vi "checkBeginNormalDefensiveWithDuelistPlay.vi"(10 "Game":refnum<class "Game.lvclass">, 11 "NormalDefensiveWithDuelistPlay in":refnum<class "NormalDefensiveWithDuelistPlay.lvclass">) -> (2 "Duelist?":bool, 3 "NormalDefensiveWithDuelistPlay out":refnum<class "NormalDefensiveWithDuelistPlay.lvclass">)   [LabVIEW 2023, in "NormalDefensiveWithDuelistPlay.lvclass"]
uses:
  NormalDefensiveWithDuelistPlay.lvclass
  Game_class/Game.lvclass
  Utilities_class/Utilities.lvclass
  Referee_class/command_interpreted.ctl
  Game_class/Game.lvclass/Game.ctl
  Ball_class/Ball.lvclass/Ball.ctl
  Object_class/Object.lvclass/Object.ctl
  Team_class/Team.lvclass/Team.ctl
  Events_class/Events.lvclass/Events.ctl
  Referee_class/Referee.lvclass/Referee.ctl
  Parameters_class/Parameters.lvclass/Parameters.ctl
  Game_class/Read Parameters.lvclass.vi
  Parameters_class/Read AttakingOurselves.vi
  Game_class/Read EventsRef.vi
  Game_class/Read Referee.vi
  Game_class/Read EnemyRef.vi
  Game_class/Read BallRef.vi
  Object_class/Read x.vi
  Object_class/Read y.vi
  Team_class/Read RobotRef.vi
  Referee_class/Read command_interpreted.vi
  Events_class/Read ball_inside_our_goalie_area.vi
  Game_class/Read OffensiveTeam.vi
  Game_class/Read FieldRef.vi
  Game_class/Read DefensiveTeam.vi
  Ball_class/Read v_x.vi
  Ball_class/Read v_y.vi
  Ball_class/Ball.lvclass
  C:/Users/roboi/Downloads/VSS_AI-Larc2023 - Copia (2)/Object_class/Object.lvclass
  Enemy_class/Enemy.lvclass
  C:/Users/roboi/Downloads/VSS_AI-Larc2023 - Copia (2)/Team_class/Team.lvclass
  Ally_class/Ally.lvclass
  Robot_class/Robot.lvclass
  Events_class/Events.lvclass
  Referee_class/Referee.lvclass
  Parameters_class/Parameters.lvclass
  Field_class/Field.lvclass
panel:
  out "error out":errorcluster
  in  "error in (no error)":errorcluster
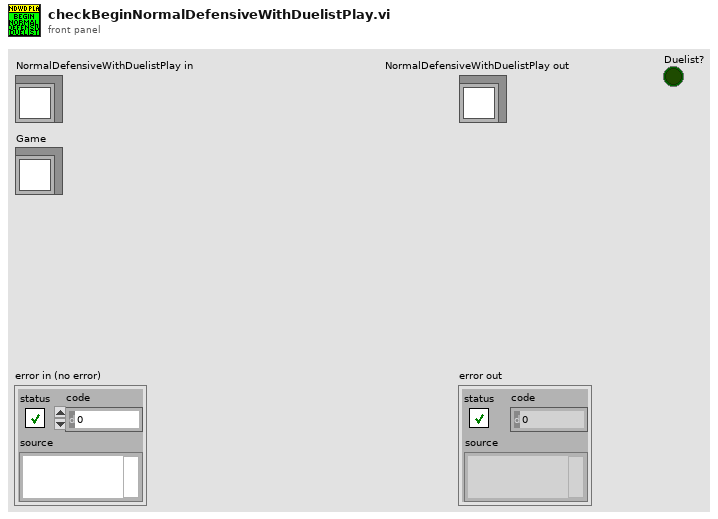
[diagram p1: front panel]
types:
  T1 = typedef "command_interpreted.ctl" = enum16{"Goal Ally", "Goal Enemy", "Ball Placement Enemy", "Ball Placement Ally", "Normal Half Time", "Extra Time  Break", "Extra Half Time", "None", "Post Game", "PKA Normal Start", "Prepare Kickoff Ally", "PKE Normal Start", "Prepare Kickoff Enemy", "Force Start", "Halt", "Timeout", "Prepare Penalty Ally", "Prepare Penalty Enemy", "PPA NormalStart", "PPE Normal Start", "Indirect Free Ally", "Direct Free Enemy", "Direct Free Ally", "Indirect Free Enemy", "Stop"}
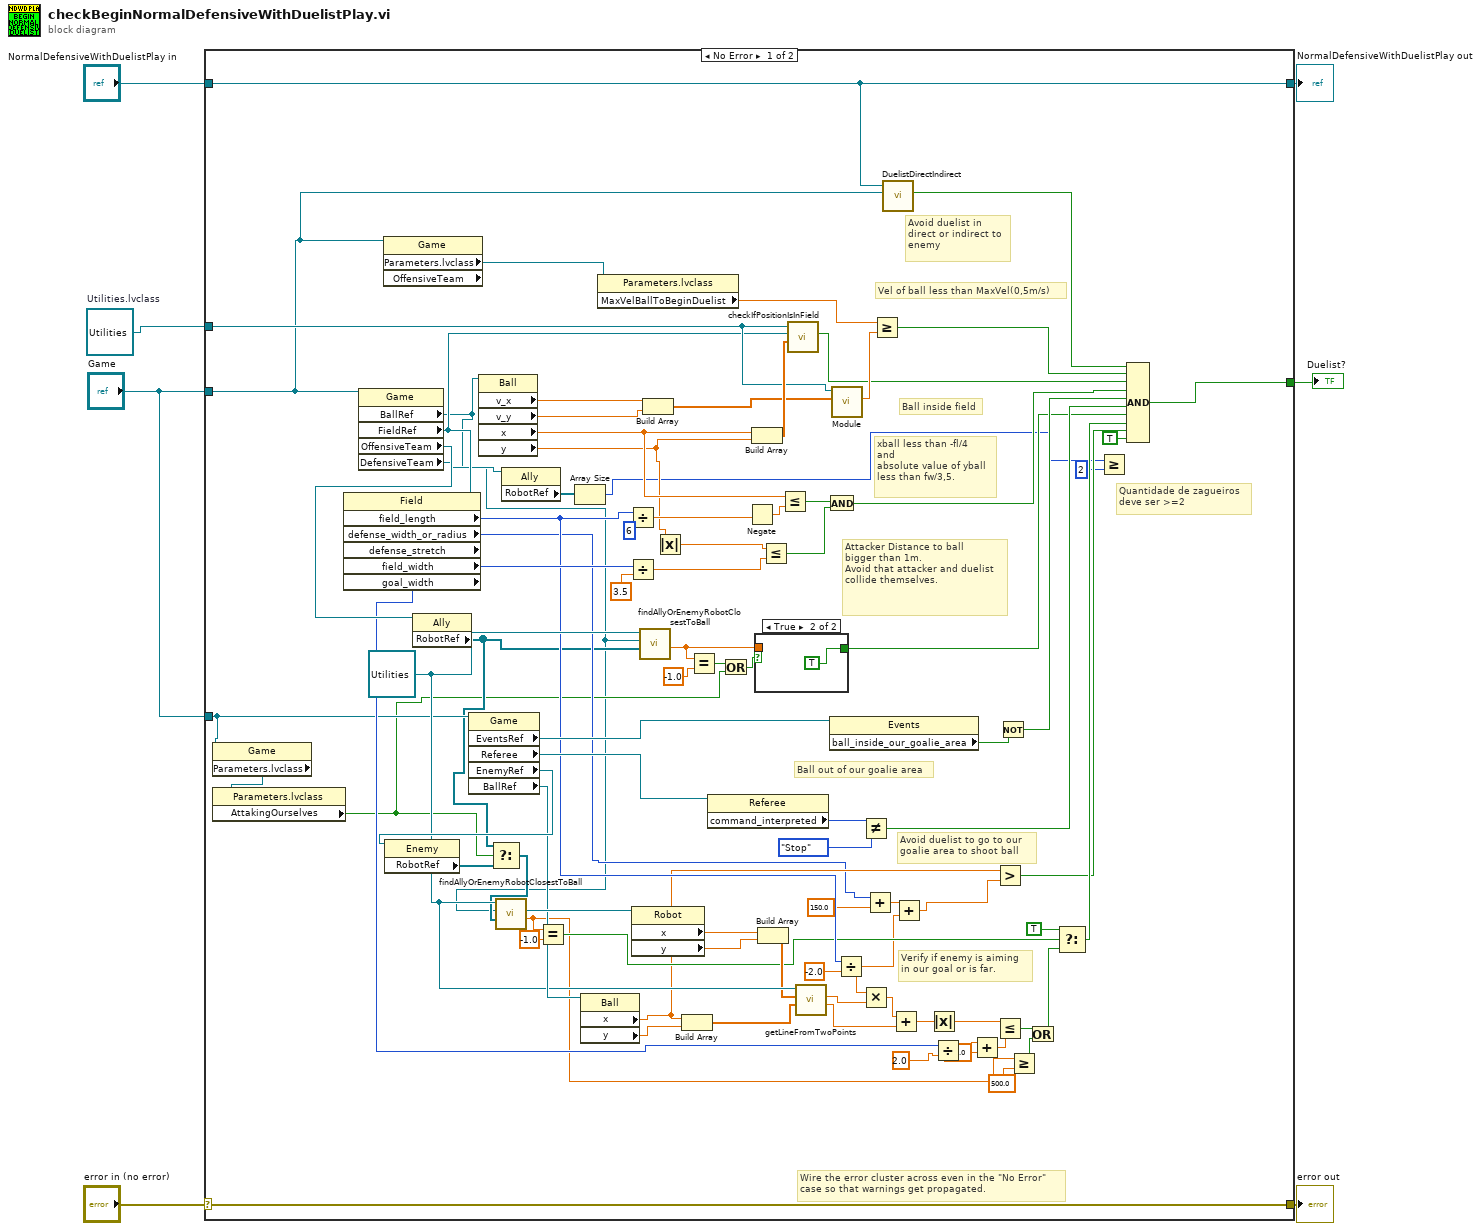
[diagram p0: block diagram]
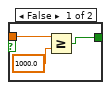
[diagram p2: hidden frame]
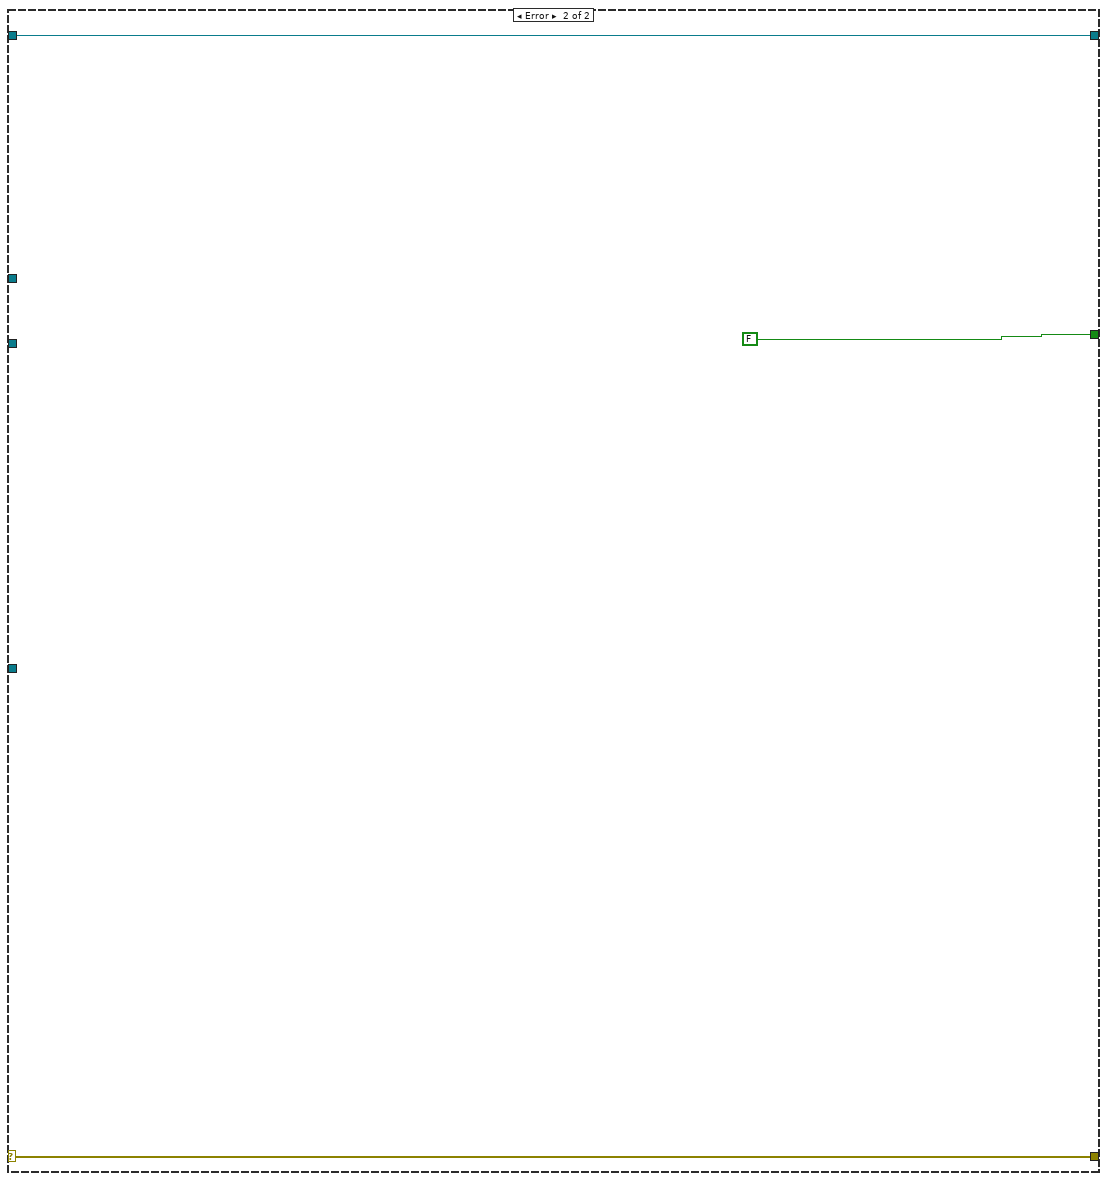
[diagram p3: hidden frame]
diagram:
  w3 = refnum<class "Utilities.lvclass"> refnum  # Utilities.lvclass
  n1 = case shown="No Error" "error in (no error)" {
    selector: "error in (no error)" -> [w97 w104]
    tunnel: [w97 w104] -> w6
    tunnel: [w83 w103] -> w4
    tunnel: "NormalDefensiveWithDuelistPlay in" -> [w83 w103]
    tunnel: w3 -> [w88 _]
    tunnel: "Game" -> [w82 _]
    tunnel: [w84 FALSE] -> w2
    tunnel: "Game" -> [w29 _]
    frame No Error {
      w54 = refnum<class "Utilities.lvclass"> refnum ("Utilities in")
      # "Quantidade de zagueiros\ndeve ser >=2"
      # "Avoid duelist to go to our\ngoalie area to shoot ball"
      # "Avoid duelist in\ndirect or indirect to\nenemy"
      # "Verify if enemy is aiming\nin our goal or is far."
      # "Attacker Distance to ball\nbigger than 1m. \nAvoid that attacker and duelist\ncollide themselves."
      # "Vel of ball less than MaxVel(0,5m/s)"
      # "Ball inside field"
      # "xball less than -fl/4\nand \nabsolute value of yball\nless than fw/3,5."
      # "Ball out of our goalie area"
      # "Wire the error cluster across even in the \"No Error\"\ncase so that warnings get propagated."
      n2 = property class="Game"(reference=w29) -> ("Parameters.lvclass"=w28:refnum<class "Parameters.lvclass">)  [unwired: 1 in, 2 out]
      n3 = property class="Parameters.lvclass"(reference=w28) -> ("AttakingOurselves"=w23:bool)  [unwired: 1 in, 2 out]
      n4 = property class="Game"(reference=w82) -> ("BallRef"=w8:refnum<class "Ball.lvclass">, "FieldRef"=w14:refnum<class "Field.lvclass">, "OffensiveTeam"=w63:refnum<class "Ally.lvclass">, "DefensiveTeam"=w13:refnum<class "Ally.lvclass">)  [unwired: 1 in, 2 out]
      n5 = property class="Field" props=["field_length", "defense_width_or_radius", "defense_stretch", "field_width", "goal_width"](reference=w14) -> ("field_length"=w48:i32, "defense_width_or_radius"=w33:i32, "field_width"=w67:i32, "goal_width"=w44:i32)  [unwired: 1 in, 3 out]
      n6 = property class="Game" props=["Parameters.lvclass", "OffensiveTeam"](reference=w82) -> ("Parameters.lvclass"=w94:refnum<class "Parameters.lvclass">)  [unwired: 1 in, 3 out]
      n7 = property class="Ally"(reference=w63) -> ("RobotRef"=w26:refnum<class "Robot.lvclass">[])  [unwired: 1 in, 2 out]
      n8 = property class="Game"(reference=w29) -> ("EventsRef"=w80:refnum<class "Events.lvclass">, "Referee"=w79:refnum<class "Referee.lvclass">, "EnemyRef"=w59:refnum<class "Enemy.lvclass">, "BallRef"=w56:refnum<class "Ball.lvclass">)  [unwired: 1 in, 2 out]
      n9 = property class="Enemy"(reference=w59) -> ("RobotRef"=w27:refnum<class "Robot.lvclass">[])  [unwired: 1 in, 2 out]
      n10 = property class="Ball"(reference=w8) -> ("v_x"=w93:dbl, "v_y"=w92:dbl, "x"=w75:dbl, "y"=w70:dbl)  [unwired: 1 in, 2 out]
      n11 = Select(t=w26, s=w23, f=w27) -> (s? t:f=w25:refnum<class "Robot.lvclass">[])
      n12 = call "findAllyOrEnemyRobotClosestToBall.vi"("Ally/Enemy Robots"=w25, "Ball"=w8, "Utilities in"=w54) -> ("Robot distance to ball"=w19:dbl, "Robot"=w58:refnum<class "Robot.lvclass">)  [unwired: 5 in, 2 out]
      n13 = property class="Ally"(reference=w13) -> ("RobotRef"=w12:refnum<class "Robot.lvclass">[])  [unwired: 1 in, 2 out]
      n14 = Equal?(x=w19, y=-1.0) -> (x = y?=w38:bool)
      n15 = Array Size(array=w12) -> (size(s)=w11:i32)
      n16 = property class="Ball"(reference=w56) -> ("x"=w36:dbl, "y"=w55:dbl)  [unwired: 1 in, 2 out]
      n17 = property class="Parameters.lvclass"(reference=w94) -> ("MaxVelBallToBeginDuelist"=w91:dbl)  [unwired: 1 in, 2 out]
      n18 = Divide(x=w48, y=6) -> (x/y=w73:dbl)
      n19 = Divide(x=w67, y=3.5) -> (x/y=w66:dbl)
      n20 = property class="Robot"(reference=w58) -> ("x"=w35:dbl, "y"=w57:dbl)  [unwired: 1 in, 2 out]
      n21 = call "findAllyOrEnemyRobotClosestToBall.vi"("Ally/Enemy Robots"=w26, "Ball"=w8, "Utilities in"=w54) -> ("Robot distance to ball"=w61:dbl)  [unwired: 5 in, 3 out]
      n22 = Build Array(w93, w92) -> (w90:dbl[])
      n23 = Absolute Value(x=w70) -> (abs(x)=w69:dbl)
      n24 = Build Array(w36, w55) -> (w52:dbl[])
      n25 = Equal?(x=w61, y=-1.0) -> (x = y?=w24:bool)
      n26 = property class="Referee"(reference=w79) -> ("command_interpreted"=w78:T1)  [unwired: 1 in, 2 out]
      n27 = Or(x=w24, y=w23) -> (x .or. y?=w22:bool)
      n28 = Negate(x=w73) -> (-x=w72:dbl)
      n29 = Build Array(w75, w70) -> (w95:dbl[])
      n30 = case shown="True" w22 {
        tunnel: w61 -> [w100 _]
        tunnel: [w98 TRUE] -> w62
        frame False {
          n31 = Greater Or Equal?(x=w100, y=1000.0) -> (x >= y?=w98:bool)
        }
        frame True {
        }
      }
      n32 = Build Array(w35, w57) -> (w53:dbl[])
      n33 = Less Or Equal?(x=w69, y=w66) -> (x <= y?=w65:bool)
      n34 = Less Or Equal?(x=w75, y=w72) -> (x <= y?=w71:bool)
      n35 = call "checkIfPositionIsInField.vi"("Position"=w95, "FieldRef"=w14, "Utilities in"=w88) -> ("Position Is In Field?"=w86:bool)  [unwired: 4 in, 4 out]
      n36 = call "getLineFromTwoPoints.vi"("Point 2"=w52, "Point 1"=w53, "Utilities in"=w54) -> ("linear coef"=w50:dbl, "angular coef"=w49:dbl)  [unwired: 4 in, 3 out]
      n37 = And(x=w71, y=w65) -> (x .and. y?=w64:bool)
      n38 = property class="Events"(reference=w80) -> ("ball_inside_our_goalie_area"=w96:bool)  [unwired: 1 in, 2 out]
      n39 = call "Module.vi"("2D vector"=w90, "Utilities in"=w88) -> ("Modulo"=w89:dbl)  [unwired: 7 in, 2 out]
      n40 = Divide(x=w48, y=-2.0) -> (x/y=w31:dbl)
      n41 = Not Equal?(x=w78, y=command_interpreted."Stop") -> (x != y?=w76:bool)
      n42 = Multiply(x=w31, y=w49) -> (x*y=w51:dbl)
      n43 = Add(x=w33, y=150.0) -> (x+y=w32:dbl)
      n44 = Greater Or Equal?(x=w91, y=w89) -> (x >= y?=w87:bool)
      n45 = call-dynamic "DuelistDirectIndirect.vi"("Game in"=w82, "NormalDefensiveWithDuelistPlay in"=w83) -> ("duelist ?"=w81:bool)  [unwired: 7 in, 2 out]
      n46 = Add(x=w51, y=w50) -> (x+y=w46:dbl)
      n47 = Add(x=w32, y=w31) -> (x+y=w30:dbl)
      n48 = Absolute Value(x=w46) -> (abs(x)=w45:dbl)
      n49 = Divide(x=w44, y=2.0) -> (x/y=w41:dbl)
      n50 = Add(x=w41, y=500.0) -> (x+y=w42:dbl)
      n51 = Greater?(x=w36, y=w30) -> (0:w15:bool)
      n52 = Less Or Equal?(x=w45, y=w42) -> (x <= y?=w21:bool)
      n53 = Not(x=w96) -> (.not. x?=w85:bool)
      n54 = Greater Or Equal?(x=w19, y=500.0) -> (x >= y?=w20:bool)
      n55 = Or(x=w21, y=w20) -> (x .or. y?=w16:bool)
      n56 = Select(t=TRUE, s=w38, f=w16) -> (s? t:f=w37:bool)
      n57 = Greater Or Equal?(x=w11, y=2) -> ()  [unwired: 1 out]
      n58 = Compound Arithmetic op=AND(w81, w87, w86, w64, w85, w76, w62, w37, w15, TRUE ("value")) -> (w84:bool)
    }
    frame Error {
    }
  }
  "error out" <- w6
  "NormalDefensiveWithDuelistPlay out" <- w4
  "Duelist?" <- w2
